vi "Configure Home Screen.vi"(8 "error IO":errorcluster, 11 "VISA resource name":refnum<visa-resource-name>) -> (0 "error Out":errorcluster, 3 "VISA resource Out":refnum<visa-resource-name>)   [LabVIEW 2020, in "eec EST 300.lvlib"]
doc: "SMM <status>\nSets the Home Screen setting.\nHome Screen: Set the default screen upon instrument power up.\nThere are 3 options:\n0=Perform Tests\n1=Menu\n2=My Menu"
uses:
  <instrlib>/eec EST 300/eec EST 300.lvlib
panel:
  in  "Home Screen":u16(ring) items=["Perform Tests", "Menu", "My Menu"]
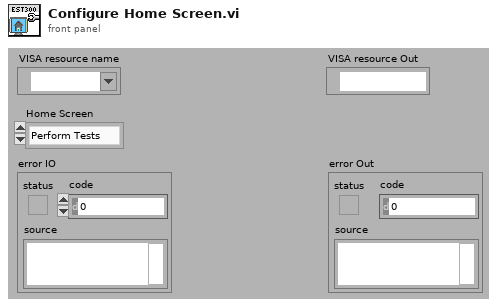
[diagram p1: front panel]
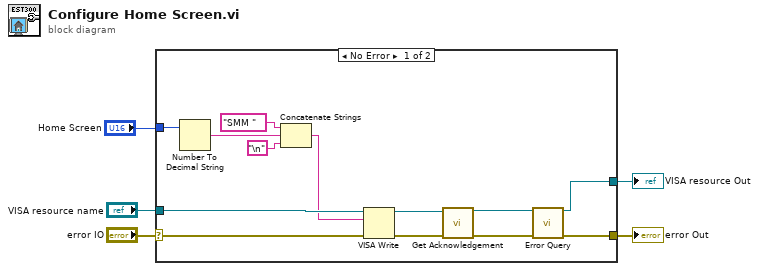
[diagram p0: block diagram]
diagram:
  n1 = case shown="No Error" "error IO" {
    selector: "error IO" -> [w18 w20]
    tunnel: [w15 w20] -> w2
    tunnel: [w16 w19] -> w3
    tunnel: "VISA resource name" -> [w17 w19]
    tunnel: "Home Screen" -> [w9 _]
    frame No Error {
      n2 = Number To Decimal String(number=w9) -> (decimal integer string=w8:string)  [unwired: 1 in]
      n3 = Concatenate Strings("SMM " ("Command to Send (empty)"), w8, "\n") -> (w12:string)
      n4 = VISA Write(VISA resource name=w17, write buffer=w12, error in (no error)=w18) -> (VISA resource name out=w6:refnum<visa-resource-name>, error out=w7:errorcluster)  [unwired: 1 out]
      n5 = call <instrlib>:"Get Acknowledgement.vi"("VISA resource name"=w6, "error in (no error)"=w7) -> ("VISA resource name out"=w11:refnum<visa-resource-name>, "error out"=w10:errorcluster)  [unwired: 12 in]
      n6 = call <instrlib>:"Error Query.vi"("VISA resource name"=w11, "error in (no error)"=w10) -> ("VISA resource name out"=w16:refnum<visa-resource-name>, "error out"=w15:errorcluster)  [unwired: 10 in, 2 out]
    }
    frame Error {
    }
  }
  "VISA resource Out" <- w3
  "error Out" <- w2
